vi "SVL Integration.vi"   [LabVIEW 2017, in "SoundVib_Integration.lvlib"]
doc: "Converts acceleration to velocity or displacement using a time-domain waveform as the input. Wire data to the <B>scaled signal [EU]</B> input to determine the polymorphic instance to use or manually select the instance."
uses:
  <vilib>/addons/Sound and Vibration/svt_Integration/SoundVib_Integration.lvlib
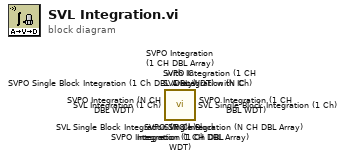
[diagram p0: block diagram]
diagram:
  n1 = call <vilib>:"SVPO Single Block Integration (1 Ch DBL WDT).vi"() -> ()  [unwired: 11 in, 1 out]
  n2 = call <vilib>:"SVPO Integration (1 CH DBL WDT) with IC.vi"() -> ()  [unwired: 10 in, 2 out]
  n3 = call <vilib>:"SVPO Integration (N CH DBL WDT).vi"() -> ()  [unwired: 11 in, 1 out]
  n4 = call <vilib>:"SVPO Integration (1 CH DBL WDT).vi"() -> ()  [unwired: 11 in, 1 out]
  n5 = call <vilib>:"SVPO Single Block Integration (1 Ch DBL Array).vi"() -> ()  [unwired: 11 in, 1 out]
  n6 = call <vilib>:"SVPO Integration (1 CH DBL Array) with IC.vi"() -> ()  [unwired: 10 in, 2 out]
  n7 = call <vilib>:"SVPO Integration (N CH DBL Array).vi"() -> ()  [unwired: 11 in, 1 out]
  n8 = call <vilib>:"SVPO Integration (1 CH DBL Array).vi"() -> ()  [unwired: 11 in, 1 out]
  n9 = call <vilib>:"SVL Single Block Integration (N Ch).vi"() -> ()  [unwired: 9 in, 3 out]
  n10 = call <vilib>:"SVL Single Block Integration (1 Ch).vi"() -> ()  [unwired: 9 in, 3 out]
  n11 = call <vilib>:"SVL Integration (1 Ch).vi"() -> ()  [unwired: 9 in, 3 out]
  n12 = call <vilib>:"SVL Integration (N Ch).vi"() -> ()  [unwired: 9 in, 3 out]
